vi "MaxiGauge_Global.vi"() -> ()   [LabVIEW 2019]
panel:
  out "MG_P5":dbl
  out "MG_P4":dbl
  out "MG_P3":dbl
  out "MG_P2":dbl
  out "MG_ST":u32(colorbox)
  out "MG_P1":dbl
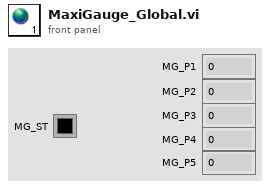
[diagram p1: front panel]
diagram:
